vi "write.vi"(8 "error in (no error)":errorcluster, 10 "writeString":string, 11 "SerialCommunicator in":refnum<class "SerialCommunicator.lvclass">) -> (0 "error out":errorcluster, 3 "SerialCommunicator out":refnum<class "SerialCommunicator.lvclass">)   [LabVIEW 2012, in "SerialProtocols.lvlib" / "SerialCommunicator.lvclass"]
uses:
  SerialCommunicator.lvclass
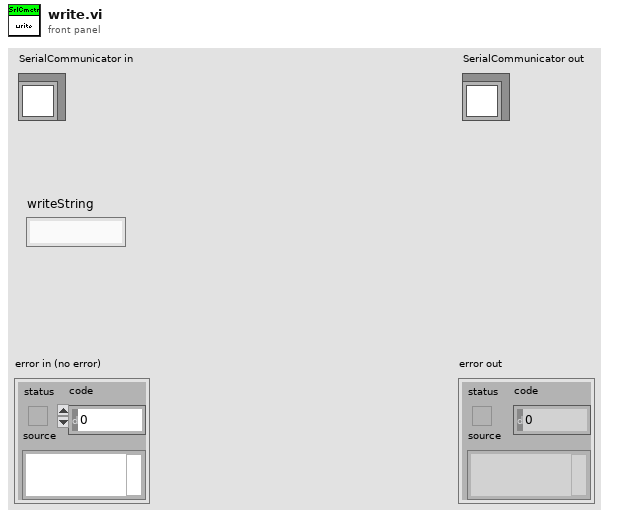
[diagram p1: front panel]
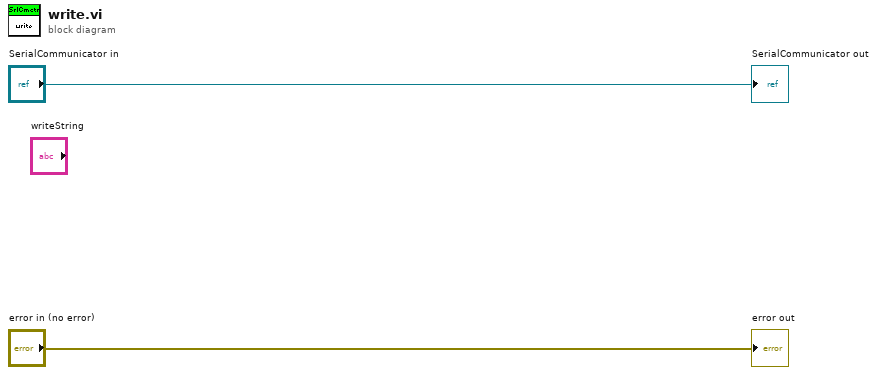
[diagram p0: block diagram]
diagram:
  "error out" <- "error in (no error)"
  "SerialCommunicator out" <- "SerialCommunicator in"
